vi "Subvi counter.vi"(0 "Reset":bool, 1 "Nmax":u64) -> (8 "Trigger":bool)   [LabVIEW 2017]
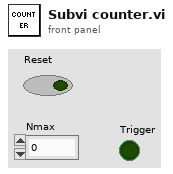
[diagram p1: front panel]
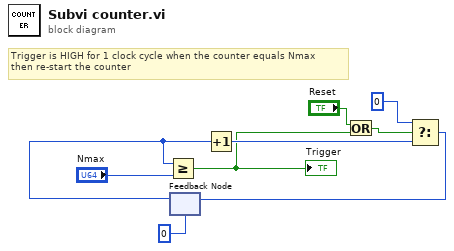
[diagram p0: block diagram]
diagram:
  # "Trigger is HIGH for 1 clock cycle when the counter equals Nmax\nthen re-start the counter"
  n1 = feedback #1(u64 0 ("t")) -> (w6:u64)
  n2 = Greater Or Equal?(x=w6, y="Nmax") -> (x >= y?=w1:bool)
  "Trigger" <- w1
  n3 = Increment(x=w6) -> (x+1=w8:u64)
  n4 = Or(x="Reset", y=w1) -> (x .or. y?=w3:bool)
  n5 = Select(t=u64 0, s=w3, f=w8) -> (s? t:f=w7:u64)
  n6 = feedback-in #1(w7) -> ()
